vi "Open Status File.vi"(8 "error in (no error)":errorcluster, 10 "path":path) -> (0 "error out":errorcluster)   [LabVIEW 2015]
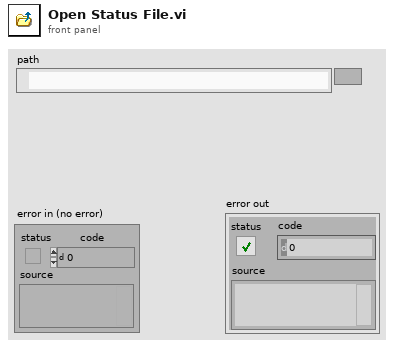
[diagram p1: front panel]
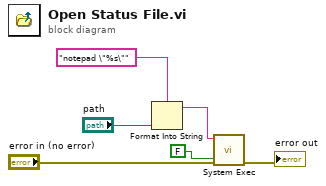
[diagram p0: block diagram]
diagram:
  n1 = Format Into String(format string="notepad \"%s\"", "path") -> (resulting string=w2:string)  [unwired: 2 in, 1 out]
  n2 = call <vilib>:"System Exec.vi"("run minimized? (F)"=FALSE, "error in (no error)"="error in (no error)", "command line"=w2) -> ("error out"=→"error out":errorcluster)  [unwired: 5 in, 3 out]
